vi "Launch Default AppBar Actor.vi"(8 "error in (no error)":errorcluster, 9 "Stop Existing? (T)":bool=TRUE, 11 "MainController in":refnum<class "MainController.lvclass">) -> (0 "error out":errorcluster, 2 "Enqueuer":refnum<class "Message Enqueuer.lvclass">, 3 "MainController out":refnum<class "MainController.lvclass">)   [LabVIEW 2012, in "Win8uiFramework.lvlib" / "MainController.lvclass"]
uses:
  MainController.lvclass
  <vilib>/ActorFramework/Message Enqueuer/Message Enqueuer.lvclass
  Visiblity States.ctl
  MainController.lvclass/MainController.ctl
  <vilib>/ActorFramework/Actor/Actor.lvclass/Actor.ctl
  <vilib>/ActorFramework/Message Enqueuer/Message Enqueuer.lvclass/Message Enqueuer.ctl
  Read Default AppBar Actor.vi
  Read AppBar Enqueuer.vi
  Write AppBar Enqueuer.vi
  Write AppBar State.vi
  <vilib>/ActorFramework/Message Enqueuer/Enqueue.vi
  <vilib>/ActorFramework/Message Enqueuer/Init from Existing Queue.vi
  <vilib>/ActorFramework/Message Priority Queue/Priority Enqueue.vi
  ViewableActor.lvclass
  <vilib>/ActorFramework/Stop Msg/Stop Msg.lvclass
  <vilib>/ActorFramework/Actor/Actor.lvclass
  Win8uiFramework.lvlib
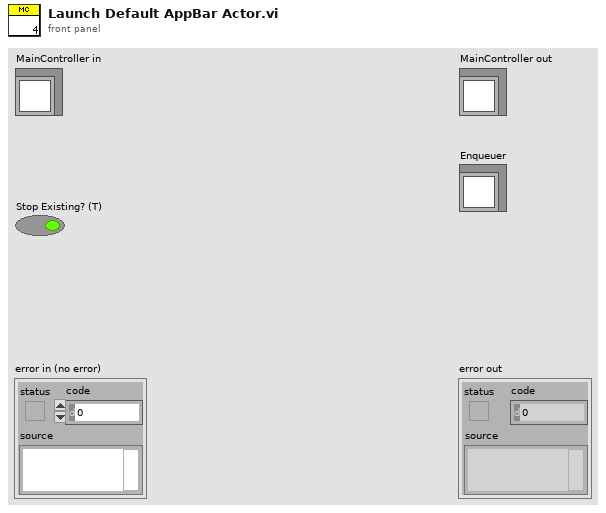
[diagram p1: front panel]
types:
  T1 = typedef "Win8uiFramework.lvlib/MainController.lvclass/Visiblity States.ctl" = enum16{"Disabled", "Hidden - Unpopulated", "Hidden - Populated", "Visible"}
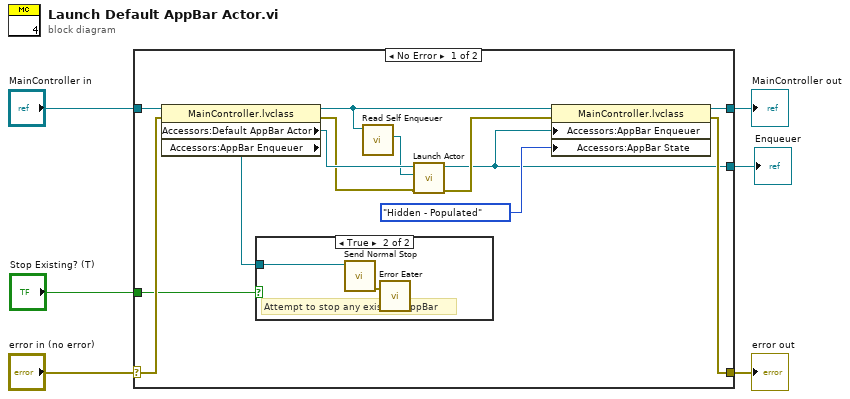
[diagram p0: block diagram]
diagram:
  n1 = case shown="No Error" "error in (no error)" {
    selector: "error in (no error)" -> [w11 w23]
    tunnel: [w10 w23] -> w5
    tunnel: [w18 w22] -> w3
    tunnel: "MainController in" -> [w19 w22]
    tunnel: [w9 _] -> w2
    tunnel: "Stop Existing? (T)" -> [w7 _]
    frame No Error {
      n2 = property class="MainController.lvclass"(reference=w19, error in=w11) -> (reference out=w17:refnum<class "MainController.lvclass">, error out=w14:errorcluster, "Accessors:Default AppBar Actor"=w16:refnum<class "ViewableActor.lvclass">, "Accessors:AppBar Enqueuer"=w8:refnum<class "Message Enqueuer.lvclass">)
      n3 = case shown="True" w7 {
        tunnel: w8 -> [_ w21]
        frame False {
        }
        frame True {
          # "Attempt to stop any existing AppBar"
          n4 = call <vilib>:"Send Normal Stop.vi"("Message Enqueuer"=w21) -> ("error out"=w20:errorcluster)  [unwired: 10 in]
          n5 = call "Error Eater.vi"("error in (no error)"=w20) -> ()  [unwired: 2 in]
        }
      }
      n6 = call <vilib>:"Read Self Enqueuer.vi"("Actor"=w17) -> ("Self Enqueuer"=w15:refnum<class "Message Enqueuer.lvclass">)  [unwired: 10 in]
      n7 = call <vilib>:"Launch Actor.vi"("error in (no error)"=w14, "Actor-to-Caller Enqueuer"=w15, "Actor"=w16) -> ("error out"=w13:errorcluster, "Caller-To-Actor Enqueuer"=w9:refnum<class "Message Enqueuer.lvclass">)  [unwired: 7 in]
      n8 = property class="MainController.lvclass"(reference=w17, error in=w13, "Accessors:AppBar Enqueuer"=w9, "Accessors:AppBar State"=Visiblity_States."Hidden - Populated" ("AppBar State")) -> (reference out=w18:refnum<class "MainController.lvclass">, error out=w10:errorcluster)
    }
    frame Error {
    }
  }
  "error out" <- w5
  "MainController out" <- w3
  "Enqueuer" <- w2
